vi "Start Command.vi"(8 "error in (no error)":errorcluster, 11 "Command in":refnum<class "Command State Actor.lvclass">) -> (0 "error out":errorcluster, 3 "Command out":refnum<class "Command State Actor.lvclass">)   [LabVIEW 2013, in "Command State Actor.lvlib" / "Command State Actor.lvclass"]
uses:
  Command State Actor.lvclass
  Command States.ctl
  Command State Actor.lvclass/Command State Actor.ctl
  Command State Messages/Go To Executing Msg/Go To Executing Msg.lvclass
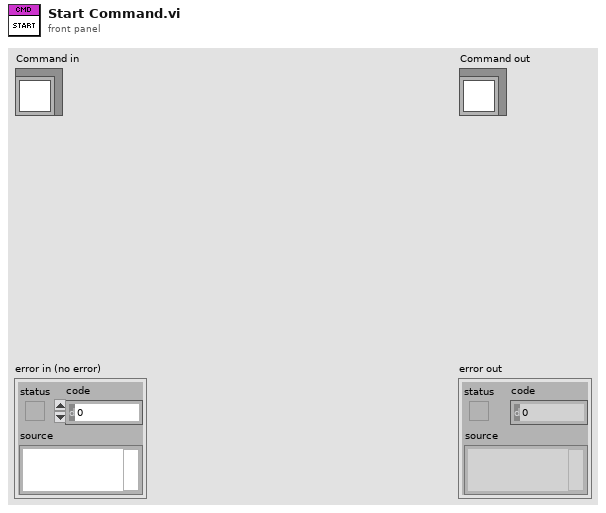
[diagram p1: front panel]
types:
  T1 = typedef "Command State Actor.lvlib/Command State Actor.lvclass/Command States.ctl" = enum16{"NotStarted", "Starting", "Started", "Executing", "Completing", "Completed", "Stopping", "Stopped"}
  T2 = typedef "Command State Actor.lvlib/Command State Actor.lvclass/Command Status.ctl" = cluster{"CurrentCommandState":T1, "Command Name":string, "Current State Status":T3, "Command Start Time":timestamp, "Command End Time":timestamp, "Previous State Status":T3}
  T3 = typedef "Command Actor.lvlib/Command States.lvclass/State Status.ctl" = cluster{"State Name":string, "State Entry Time":timestamp, "State Exit Time":timestamp}
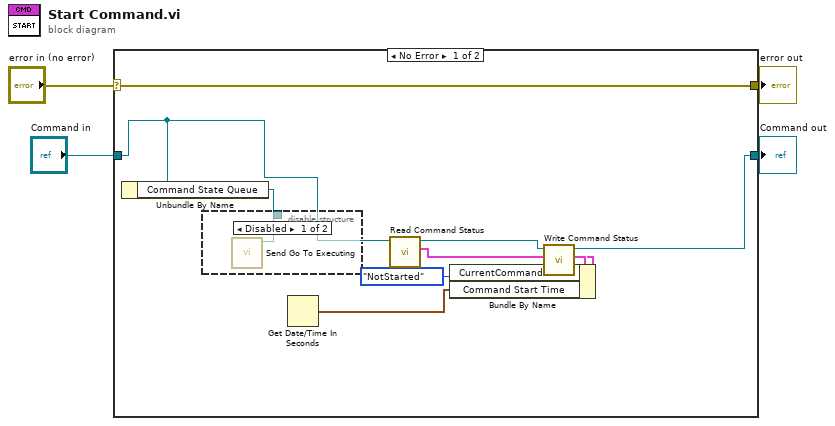
[diagram p0: block diagram]
diagram:
  n1 = case shown="No Error" "error in (no error)" {
    selector: "error in (no error)" -> [w13 w16]
    tunnel: [w13 w16] -> w3
    tunnel: [w9 w15] -> w1
    tunnel: "Command in" -> [w11 w15]
    frame No Error {
      n2 = Unbundle By Name(w11) -> ("Command State Queue"=w12:refnum<class "Message Enqueuer.lvclass">)
      n3 = disable-structure shown="Disabled" {
        disable-tunnel: w12 -> [w14 _]
        frame Disabled {
          n4 = call "Send Go To Executing.vi"("Message Enqueuer"=w14) -> ()  [unwired: 9 in, 2 out]
        }
        frame Enabled {
        }
      }
      n5 = Get Date/Time In Seconds() -> (seconds since 1Jan1904=w5:timestamp)
      n6 = call-dynamic "Read Command Status.vi"("Command in"=w11) -> ("Command Status"=w8:T2, "Command out"=w10:refnum<class "Command State Actor.lvclass">)  [unwired: 8 in, 1 out]
      n7 = Bundle By Name(cluster=w8, "CurrentCommandState"=Command_States."NotStarted", "Command Start Time"=w5) -> (w7:T2)
      n8 = call-dynamic "Write Command Status.vi"("Command Status"=w7, "Command in"=w10) -> ("Command out"=w9:refnum<class "Command State Actor.lvclass">)  [unwired: 8 in, 1 out]
    }
    frame Error {
    }
  }
  "error out" <- w3
  "Command out" <- w1
